vi "INSTRUMENTORDERSVotage.vi"(0 "VISA资源名称":refnum<visa-resource-name>="DPO5054-C012667", 1 "打开通道":u16(ring) items=["CH1", "CH2", "CH3", "CH4"], 2 "关闭通道":u16(ring) items=["CH1", "CH2", "CH3", "CH4"], 3 "行索引":i32, 5 "错误输入（无错误）":errorcluster) -> (11 "FREQ":dbl, 13 "PERIOD":dbl, 14 "RMS":dbl, 15 "AMP":dbl, 16 "MAX":dbl, 17 "MIN":dbl, 18 "PK2PK":dbl, 19 "错误输出":errorcluster)   [LabVIEW 2014]
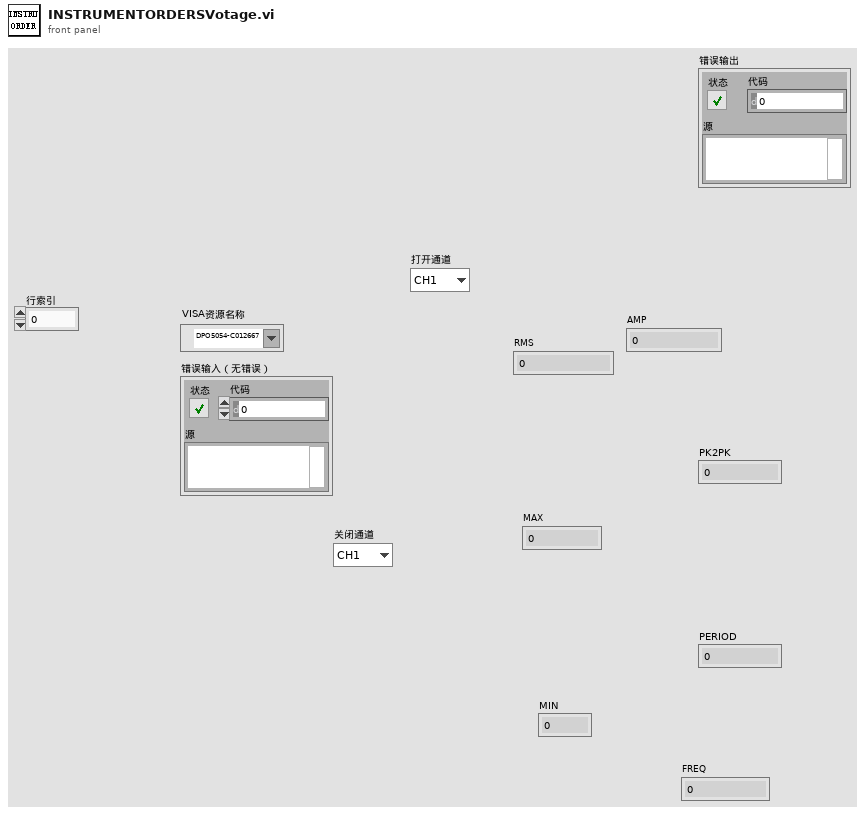
[diagram p1: front panel]
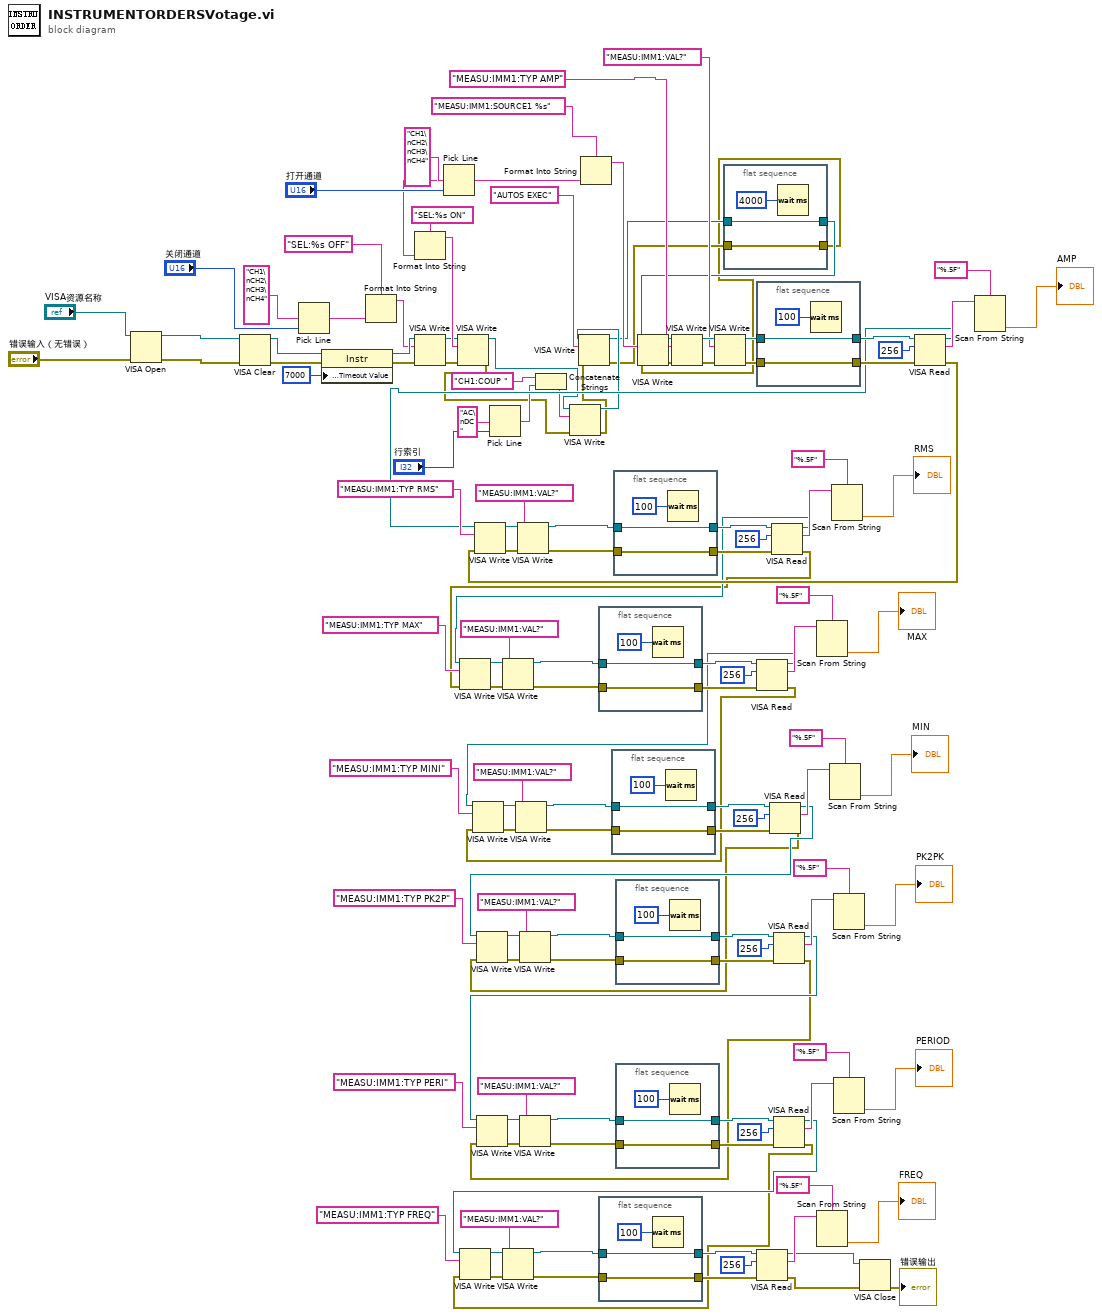
[diagram p0: block diagram]
diagram:
  n1 = VISA Open(error in (no error)="错误输入（无错误）", VISA resource name="VISA资源名称") -> (VISA resource name=w137:refnum<visa-resource-name>, error out=w136:errorcluster)  [unwired: 3 in]
  n2 = VISA Clear(VISA resource name=w137, error in (no error)=w136) -> (VISA resource name out=w135:refnum<visa-resource-name>, error out=w134:errorcluster)
  n3 = Pick Line(multi-line string="CH1\nCH2\nCH3\nCH4" ("多行字符串"), line index="关闭通道") -> (output string=w111:string)  [unwired: 1 in]
  n4 = property class="Instr"(reference=w135, error in=w134, "General Settings:Timeout Value"=u32 7000) -> (reference out=w113:refnum<visa-resource-name>, error out=w112:errorcluster)
  n5 = Format Into String(format string="SEL:%s OFF" ("格式字符串"), w111) -> (resulting string=w107:string)  [unwired: 2 in, 1 out]
  n6 = VISA Write(VISA resource name=w113, write buffer=w107, error in (no error)=w112) -> (VISA resource name out=w106:refnum<visa-resource-name>, error out=w105:errorcluster)  [unwired: 1 out]
  n7 = Pick Line(multi-line string="CH1\nCH2\nCH3\nCH4" ("多行字符串"), line index="打开通道") -> (output string=w116:string)  [unwired: 1 in]
  n8 = Format Into String(format string="SEL:%s ON" ("格式字符串"), w116) -> (resulting string=w115:string)  [unwired: 2 in, 1 out]
  n9 = VISA Write(VISA resource name=w106, write buffer=w115, error in (no error)=w105) -> (VISA resource name out=w8:refnum<visa-resource-name>, error out=w7:errorcluster)  [unwired: 1 out]
  n10 = Pick Line(multi-line string="AC\nDC", line index="行索引") -> (output string=w10:string)  [unwired: 1 in]
  n11 = Concatenate Strings("CH1:COUP " ("写入缓冲区"), w10) -> (w9:string)
  n12 = VISA Write(VISA resource name=w8, write buffer=w9, error in (no error)=w7) -> (VISA resource name out=w6:refnum<visa-resource-name>, error out=w5:errorcluster)  [unwired: 1 out]
  n13 = VISA Write(VISA resource name=w6, write buffer="AUTOS EXEC" ("写入缓冲区"), error in (no error)=w5) -> (VISA resource name out=w4:refnum<visa-resource-name>, error out=w3:errorcluster)  [unwired: 1 out]
  n14 = Format Into String(format string="MEASU:IMM1:SOURCE1 %s" ("格式字符串"), w116) -> (resulting string=w129:string)  [unwired: 2 in, 1 out]
  n15 = flat-sequence {
    tunnel: w87 -> [w140]
    tunnel: [w140] -> w85
    tunnel: w88 -> [w139]
    tunnel: [w139] -> w84
    frame #0 {
      n16 = Wait (ms)(milliseconds to wait=u32 100 ("等待时间（毫秒）")) -> ()  [unwired: 1 out]
    }
  }
  n17 = flat-sequence {
    tunnel: w39 -> [w143]
    tunnel: [w143] -> w37
    tunnel: w40 -> [w142]
    tunnel: [w142] -> w36
    frame #0 {
      n18 = Wait (ms)(milliseconds to wait=u32 100 ("等待时间（毫秒）")) -> ()  [unwired: 1 out]
    }
  }
  n19 = flat-sequence {
    tunnel: w66 -> [w146]
    tunnel: [w146] -> w68
    tunnel: w65 -> [w145]
    tunnel: [w145] -> w69
    frame #0 {
      n20 = Wait (ms)(milliseconds to wait=u32 100 ("等待时间（毫秒）")) -> ()  [unwired: 1 out]
    }
  }
  n21 = flat-sequence {
    tunnel: w90 -> [w149]
    tunnel: [w149] -> w92
    tunnel: w89 -> [w148]
    tunnel: [w148] -> w93
    frame #0 {
      n22 = Wait (ms)(milliseconds to wait=u32 100 ("等待时间（毫秒）")) -> ()  [unwired: 1 out]
    }
  }
  n23 = flat-sequence {
    tunnel: w63 -> [w152]
    tunnel: [w152] -> w61
    tunnel: w64 -> [w151]
    tunnel: [w151] -> w60
    frame #0 {
      n24 = Wait (ms)(milliseconds to wait=u32 100 ("等待时间（毫秒）")) -> ()  [unwired: 1 out]
    }
  }
  n25 = flat-sequence {
    tunnel: w42 -> [w155]
    tunnel: [w155] -> w44
    tunnel: w41 -> [w154]
    tunnel: [w154] -> w45
    frame #0 {
      n26 = Wait (ms)(milliseconds to wait=u32 100 ("等待时间（毫秒）")) -> ()  [unwired: 1 out]
    }
  }
  n27 = VISA Write(VISA resource name=w2, write buffer=w129, error in (no error)=w1) -> (VISA resource name out=w126:refnum<visa-resource-name>, error out=w125:errorcluster)  [unwired: 1 out]
  n28 = VISA Write(VISA resource name=w126, write buffer="MEASU:IMM1:TYP AMP" ("写入缓冲区"), error in (no error)=w125) -> (VISA resource name out=w122:refnum<visa-resource-name>, error out=w121:errorcluster)  [unwired: 1 out]
  n29 = VISA Write(VISA resource name=w122, write buffer="MEASU:IMM1:VAL?" ("写入缓冲区"), error in (no error)=w121) -> (VISA resource name out=w119:refnum<visa-resource-name>, error out=w118:errorcluster)  [unwired: 1 out]
  n30 = flat-sequence {
    tunnel: w4 -> [w158]
    tunnel: [w158] -> w2
    tunnel: w3 -> [w157]
    tunnel: [w157] -> w1
    frame #0 {
      n31 = Wait (ms)(milliseconds to wait=u32 4000 ("等待时间（毫秒）")) -> ()  [unwired: 1 out]
    }
  }
  n32 = flat-sequence {
    tunnel: w119 -> [w161]
    tunnel: [w161] -> w124
    tunnel: w118 -> [w160]
    tunnel: [w160] -> w123
    frame #0 {
      n33 = Wait (ms)(milliseconds to wait=u32 100 ("等待时间（毫秒）")) -> ()  [unwired: 1 out]
    }
  }
  n34 = VISA Read(VISA resource name=w85, byte count=u32 256 ("字节总数"), error in (no error)=w84) -> (VISA resource name out=w24:refnum<visa-resource-name>, read buffer=w83:string, error out=w23:errorcluster)  [unwired: 1 out]
  n35 = VISA Write(VISA resource name=w24, write buffer="MEASU:IMM1:TYP MINI" ("写入缓冲区"), error in (no error)=w23) -> (VISA resource name out=w74:refnum<visa-resource-name>, error out=w75:errorcluster)  [unwired: 1 out]
  n36 = VISA Write(VISA resource name=w74, write buffer="MEASU:IMM1:VAL?" ("写入缓冲区"), error in (no error)=w75) -> (VISA resource name out=w66:refnum<visa-resource-name>, error out=w65:errorcluster)  [unwired: 1 out]
  n37 = VISA Read(VISA resource name=w37, byte count=u32 256 ("字节总数"), error in (no error)=w36) -> (VISA resource name out=w16:refnum<visa-resource-name>, read buffer=w35:string, error out=w15:errorcluster)  [unwired: 1 out]
  n38 = VISA Read(VISA resource name=w68, byte count=u32 256 ("字节总数"), error in (no error)=w69) -> (VISA resource name out=w22:refnum<visa-resource-name>, read buffer=w70:string, error out=w21:errorcluster)  [unwired: 1 out]
  n39 = VISA Write(VISA resource name=w22, write buffer="MEASU:IMM1:TYP PK2P" ("写入缓冲区"), error in (no error)=w21) -> (VISA resource name out=w55:refnum<visa-resource-name>, error out=w54:errorcluster)  [unwired: 1 out]
  n40 = VISA Write(VISA resource name=w55, write buffer="MEASU:IMM1:VAL?" ("写入缓冲区"), error in (no error)=w54) -> (VISA resource name out=w63:refnum<visa-resource-name>, error out=w64:errorcluster)  [unwired: 1 out]
  n41 = VISA Read(VISA resource name=w92, byte count=u32 256 ("字节总数"), error in (no error)=w93) -> (VISA resource name out=w26:refnum<visa-resource-name>, read buffer=w94:string, error out=w25:errorcluster)  [unwired: 1 out]
  n42 = VISA Write(VISA resource name=w26, write buffer="MEASU:IMM1:TYP MAX" ("写入缓冲区"), error in (no error)=w25) -> (VISA resource name out=w79:refnum<visa-resource-name>, error out=w78:errorcluster)  [unwired: 1 out]
  n43 = VISA Write(VISA resource name=w79, write buffer="MEASU:IMM1:VAL?" ("写入缓冲区"), error in (no error)=w78) -> (VISA resource name out=w87:refnum<visa-resource-name>, error out=w88:errorcluster)  [unwired: 1 out]
  n44 = VISA Read(VISA resource name=w61, byte count=u32 256 ("字节总数"), error in (no error)=w60) -> (VISA resource name out=w20:refnum<visa-resource-name>, read buffer=w59:string, error out=w19:errorcluster)  [unwired: 1 out]
  n45 = VISA Write(VISA resource name=w20, write buffer="MEASU:IMM1:TYP PERI" ("写入缓冲区"), error in (no error)=w19) -> (VISA resource name out=w50:refnum<visa-resource-name>, error out=w51:errorcluster)  [unwired: 1 out]
  n46 = VISA Write(VISA resource name=w50, write buffer="MEASU:IMM1:VAL?" ("写入缓冲区"), error in (no error)=w51) -> (VISA resource name out=w42:refnum<visa-resource-name>, error out=w41:errorcluster)  [unwired: 1 out]
  n47 = VISA Read(VISA resource name=w44, byte count=u32 256 ("字节总数"), error in (no error)=w45) -> (VISA resource name out=w18:refnum<visa-resource-name>, read buffer=w46:string, error out=w17:errorcluster)  [unwired: 1 out]
  n48 = VISA Write(VISA resource name=w18, write buffer="MEASU:IMM1:TYP FREQ" ("写入缓冲区"), error in (no error)=w17) -> (VISA resource name out=w31:refnum<visa-resource-name>, error out=w30:errorcluster)  [unwired: 1 out]
  n49 = VISA Write(VISA resource name=w31, write buffer="MEASU:IMM1:VAL?" ("写入缓冲区"), error in (no error)=w30) -> (VISA resource name out=w39:refnum<visa-resource-name>, error out=w40:errorcluster)  [unwired: 1 out]
  n50 = Scan From String(format string="%.5F" ("格式字符串"), input string=w83) -> (output 1=→"MAX":dbl)  [unwired: 3 in, 3 out]
  n51 = Scan From String(format string="%.5F" ("格式字符串"), input string=w35) -> (output 1=→"FREQ":dbl)  [unwired: 3 in, 3 out]
  n52 = Scan From String(format string="%.5F" ("格式字符串"), input string=w70) -> (output 1=→"MIN":dbl)  [unwired: 3 in, 3 out]
  n53 = Scan From String(format string="%.5F" ("格式字符串"), input string=w94) -> (output 1=→"RMS":dbl)  [unwired: 3 in, 3 out]
  n54 = Scan From String(format string="%.5F" ("格式字符串"), input string=w59) -> (output 1=→"PK2PK":dbl)  [unwired: 3 in, 3 out]
  n55 = Scan From String(format string="%.5F" ("格式字符串"), input string=w46) -> (output 1=→"PERIOD":dbl)  [unwired: 3 in, 3 out]
  n56 = VISA Close(VISA resource name=w16, error in (no error)=w15) -> (error out=→"错误输出":errorcluster)
  n57 = VISA Read(VISA resource name=w124, byte count=u32 256 ("字节总数"), error in (no error)=w123) -> (VISA resource name out=w28:refnum<visa-resource-name>, read buffer=w103:string, error out=w27:errorcluster)  [unwired: 1 out]
  n58 = VISA Write(VISA resource name=w28, write buffer="MEASU:IMM1:TYP RMS" ("写入缓冲区"), error in (no error)=w27) -> (VISA resource name out=w98:refnum<visa-resource-name>, error out=w99:errorcluster)  [unwired: 1 out]
  n59 = VISA Write(VISA resource name=w98, write buffer="MEASU:IMM1:VAL?" ("写入缓冲区"), error in (no error)=w99) -> (VISA resource name out=w90:refnum<visa-resource-name>, error out=w89:errorcluster)  [unwired: 1 out]
  n60 = Scan From String(format string="%.5F" ("格式字符串"), input string=w103) -> (output 1=→"AMP":dbl)  [unwired: 3 in, 3 out]
